vi "Get Measurement Details.vi"(8 "error in":errorcluster) -> (0 "error out":errorcluster, 1 "measurement annotations":T1[](array[typedef]), 2 "service class":string, 3 "measurement details":T2)   [LabVIEW 2021, in "Full Scale Error_ADC.lvlib"]
uses:
  Full Scale Error_ADC.lvlib
  <vilib>/Plug-In SDKs/Measurements/NI Measurement Plug-In SDK.lvlib
  <vilib>/gRPC/Generated APIs/ni/measurementlink/measurement/v1/RPC Messages/ni_measurementlink_measurement_v1_MeasurementDetails.ctl
  <vilib>/gRPC/Generated APIs/ni/measurementlink/measurement/v1/ni.measurementlink.measurement.v1.api.lvlib
  <vilib>/Plug-In SDKs/Measurements/Helpers/TypeDefs/Measurement Annotation.ctl
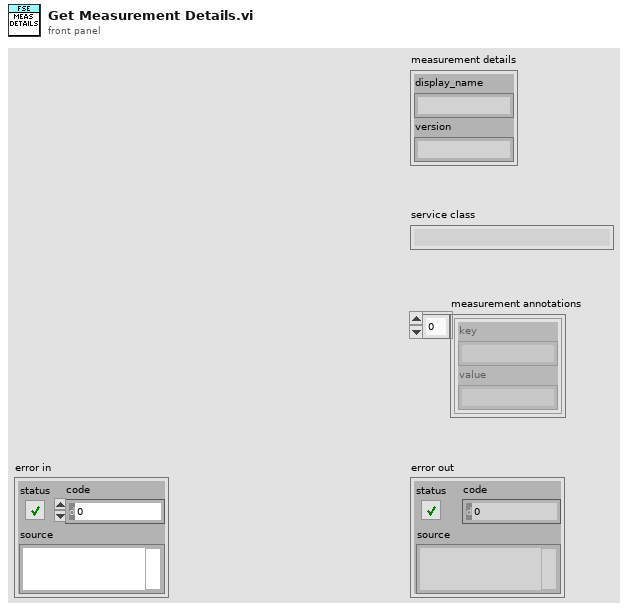
[diagram p1: front panel]
types:
  T1 = typedef "NI Measurement Plug-In SDK.lvlib/Measurement Annotation.ctl" = cluster{"key":string, "value":string}
  T2 = typedef "ni.measurementlink.measurement.v1.api.lvlib/ni_measurementlink_measurement_v1_MeasurementDetails.ctl" = cluster{"display_name":string, "version":string}
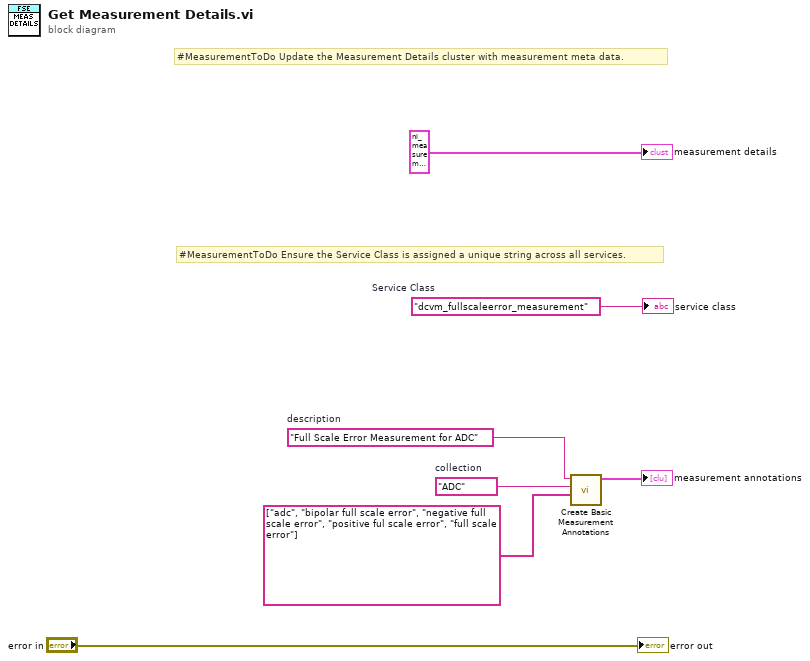
[diagram p0: block diagram]
diagram:
  w2 = "ADC"  # collection
  w3 = "Full Scale Error Measurement for ADC"  # description
  w6 = "dcvm_fullscaleerror_measurement"  # Service Class
  # "#MeasurementToDo Ensure the Service Class is assigned a unique string across all services."
  # "#MeasurementToDo Update the Measurement Details cluster with measurement meta data."
  n1 = call <vilib>:"Create Basic Measurement Annotations.vi"("tags"=string[] ["adc", "bipolar full scale error", "negative full scale error", "positive ful scale error", "full scale error"], "collection"=w2, "description"=w3) -> ("measurement annotations"=→"measurement annotations":T1[])  [unwired: 7 in, 1 out]
  "error out" <- "error in"
  "measurement details" <- T2 {"display_name"="DCVM - Full Scale Error Measurement", "version"="2.0.0"} ("Measurement Details")
  "service class" <- w6
